vi "THETA_1.vi"(8 "error in (no error)":errorcluster, 11 "reference in":refnum<class "Manipulator.lvclass">) -> (0 "error out":errorcluster, 2 "THETA_1":dbl, 3 "reference out":refnum<class "Manipulator.lvclass">)   [LabVIEW 2014, in "Manipulator.lvclass"]
uses:
  Manipulator.lvclass
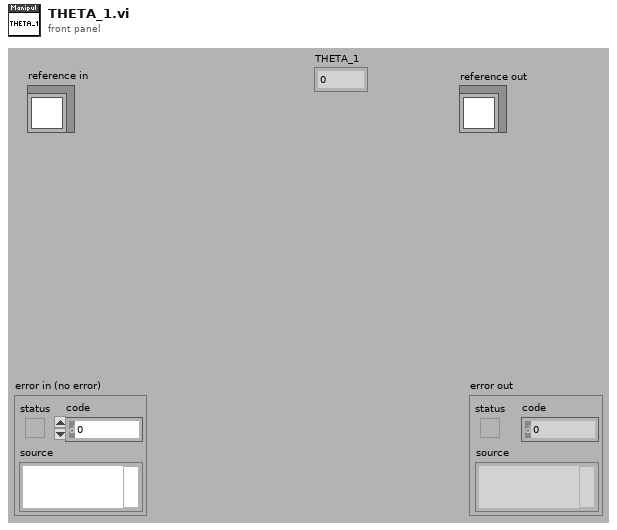
[diagram p1: front panel]
types:
  T1 = typedef "Manipulator.lvclass/ObjectAttributes.ctl" = cluster{"Coordinates":cluster{"X":dbl, "Y":dbl, "Z":dbl}, "Angles":cluster{"THETA_1":dbl, "THETA_2":dbl, "THETA_3":dbl, "THETA_4":dbl, "THETA_5":dbl, "THETA_6":dbl, "THETA_7":dbl, "THETA_8":dbl, "THETA_9":dbl, "THETA_10":dbl}, "Lengths":cluster{"a":dbl, "b":dbl, "c":dbl, "d":dbl, "e":dbl}, "Coordinates of joints":cluster{"A":cluster{"X":dbl, "Y":dbl, "Z":dbl}, "B":cluster{"X":dbl, "Y":dbl, "Z":dbl}, "C":cluster{"X":dbl, "Y":dbl, "Z":dbl}, "D":cluster{"X":dbl, "Y":dbl, "Z":dbl}}}
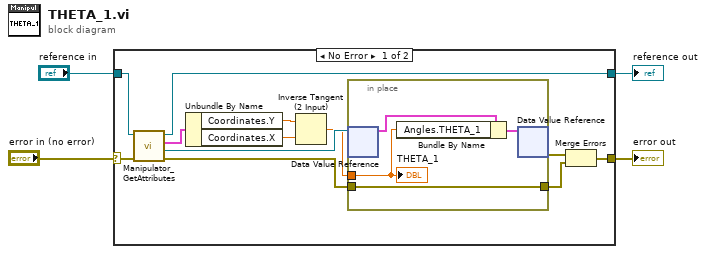
[diagram p0: block diagram]
diagram:
  n1 = case shown="No Error" "error in (no error)" {
    selector: "error in (no error)" -> [w15 w22]
    tunnel: [w11 w22] -> w3
    tunnel: [w12 w21] -> w1
    tunnel: "reference in" -> [w16 w21]
    frame No Error {
      n2 = call "Manipulator_GetAttributes.vi"("error in (no error)"=w15, "reference in"=w16) -> ("error out"=w9:errorcluster, "DataRef"=w10:refnum<data-value>, "Data"=w14:T1, "reference out"=w12:refnum<class "Manipulator.lvclass">)  [unwired: 6 in]
      n3 = Unbundle By Name(w14) -> ("Coordinates.Y"=w7:dbl, "Coordinates.X"=w6:dbl)
      n4 = Inverse Tangent (2 Input)(1:w6, 2:w7) -> (0:w5:dbl)
      n5 = in-place {
        in-place-border: w9 -> [w20]
        in-place-border: [w20] -> w8
        in-place-border: w5 -> [w18]
        n6 = in-place-dvr #1(w10) -> (w19:T1)  [unwired: 1 out]
        n7 = Bundle By Name(cluster=w19, "Angles.THETA_1"=w18) -> (w17:T1)
        n8 = in-place-dvr #1(w17) -> (w13:errorcluster)  [unwired: 1 out]
        "THETA_1" <- w18
      }
      n9 = Merge Errors(w13, w8) -> (w11:errorcluster)
    }
    frame Error {
    }
  }
  "error out" <- w3
  "reference out" <- w1
